vi "set output trigger.vi"(8 "error in (no error)":errorcluster, 11 "DAQOrcaFlash in":refnum<class "DAQOrcaFlash.lvclass">) -> (0 "error out":errorcluster, 3 "DAQOrcaFlash out":refnum<class "DAQOrcaFlash.lvclass">)   [LabVIEW 2012, in "DAQOrcaFlash.lvclass"]
uses:
  DAQOrcaFlash.lvclass
  connector.ctl
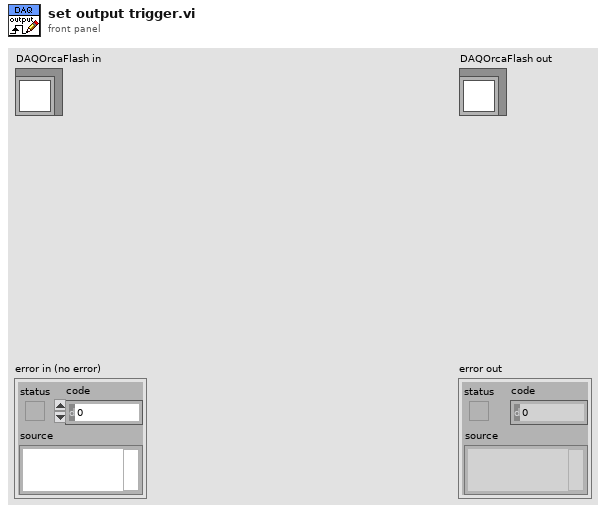
[diagram p1: front panel]
types:
  T1 = typedef "DAQOrcaFlash.lvclass/connector.ctl" = enum32{"1", "2", "3"}
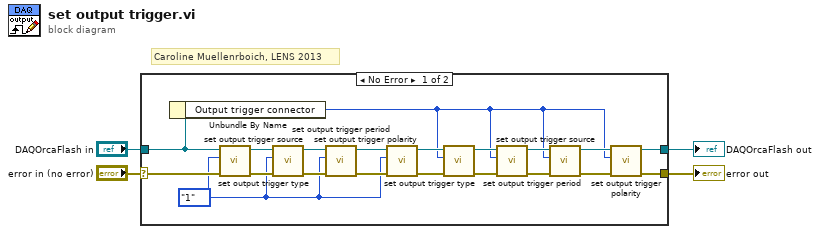
[diagram p0: block diagram]
diagram:
  # "Caroline Muellenrboich, LENS 2013"
  n1 = case shown="No Error" "error in (no error)" {
    selector: "error in (no error)" -> [w10 w26]
    tunnel: [w17 w26] -> w4
    tunnel: [w19 w25] -> w2
    tunnel: "DAQOrcaFlash in" -> [w7 w25]
    frame No Error {
      w5 = connector."1" ("Output trigger connector")
      n2 = Unbundle By Name(w7) -> ("Output trigger connector"=w6:T1)
      n3 = call-dynamic "set output trigger type.vi"("error in (no error)"=w10, "Output trigger connector"=w5, "DAQOrcaFlash in"=w7) -> ("error out"=w14:errorcluster, "DAQOrcaFlash out"=w16:refnum<class "DAQOrcaFlash.lvclass">)  [unwired: 7 in]
      n4 = call-dynamic "set output trigger source.vi"("error in (no error)"=w14, "Output trigger connector"=w5, "DAQOrcaFlash in"=w16) -> ("error out"=w13:errorcluster, "DAQOrcaFlash out"=w15:refnum<class "DAQOrcaFlash.lvclass">)  [unwired: 7 in]
      n5 = call-dynamic "set output trigger period.vi"("error in (no error)"=w13, "Output trigger connector"=w5, "DAQOrcaFlash in"=w15) -> ("error out"=w11:errorcluster, "DAQOrcaFlash out"=w12:refnum<class "DAQOrcaFlash.lvclass">)  [unwired: 7 in]
      n6 = call-dynamic "set output trigger polarity.vi"("error in (no error)"=w11, "Output trigger connector"=w5, "DAQOrcaFlash in"=w12) -> ("error out"=w9:errorcluster, "DAQOrcaFlash out"=w8:refnum<class "DAQOrcaFlash.lvclass">)  [unwired: 7 in]
      n7 = call-dynamic "set output trigger type.vi"("error in (no error)"=w9, "Output trigger connector"=w6, "DAQOrcaFlash in"=w8) -> ("error out"=w22:errorcluster, "DAQOrcaFlash out"=w24:refnum<class "DAQOrcaFlash.lvclass">)  [unwired: 7 in]
      n8 = call-dynamic "set output trigger source.vi"("error in (no error)"=w22, "Output trigger connector"=w6, "DAQOrcaFlash in"=w24) -> ("error out"=w21:errorcluster, "DAQOrcaFlash out"=w23:refnum<class "DAQOrcaFlash.lvclass">)  [unwired: 7 in]
      n9 = call-dynamic "set output trigger period.vi"("error in (no error)"=w21, "Output trigger connector"=w6, "DAQOrcaFlash in"=w23) -> ("error out"=w18:errorcluster, "DAQOrcaFlash out"=w20:refnum<class "DAQOrcaFlash.lvclass">)  [unwired: 7 in]
      n10 = call-dynamic "set output trigger polarity.vi"("error in (no error)"=w18, "Output trigger connector"=w6, "DAQOrcaFlash in"=w20) -> ("error out"=w17:errorcluster, "DAQOrcaFlash out"=w19:refnum<class "DAQOrcaFlash.lvclass">)  [unwired: 7 in]
    }
    frame Error {
    }
  }
  "error out" <- w4
  "DAQOrcaFlash out" <- w2
